vi "configureForVoltageOutput.vi"(2 "error in (no error)":errorcluster, 3 "Output Properties":T1, 4 "AnalogOutput in":refnum<class "AnalogOutput.lvclass">) -> (0 "error out":errorcluster, 1 "AnalogOutput out":refnum<class "AnalogOutput.lvclass">)   [LabVIEW 2011, in "Hardware.lvlib" / "Channels.lvlib" / "AnalogOutput.lvclass"]
doc: "Abstract Method.\n\nThis vi set the channel name, physical channel, and the output range of the DAC. It calls createChannel which is implemented by child classes (for example, niDAQmxAO).\n\nThe cluster passed to this vi includes:\n1) Name (string)\n2) Channels (String)\n3) Ranges (Double Array 1D)"
uses:
  AnalogOutput.lvclass
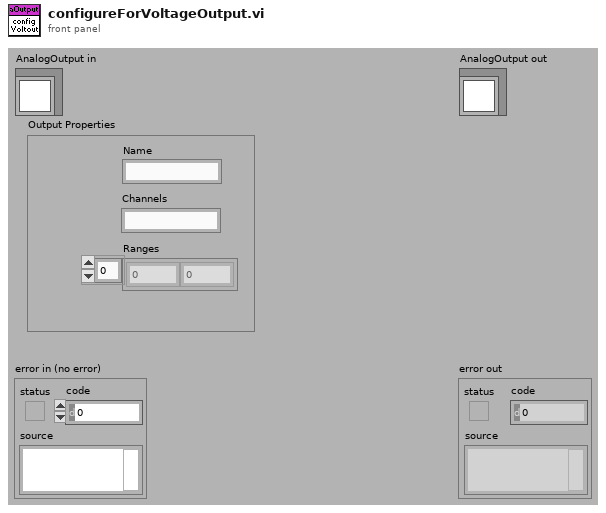
[diagram p1: front panel]
types:
  T1 = cluster{"Name":string, "Channels":string, "Ranges":dbl[]}
  T2 = cluster{"Configuration Type":cluster{"Differential":i16, "Pseudodifferential":i16, "RSE":dbl}, "Output Type":cluster{"Voltage":string, "Current":string, "Standard Function ":cluster{"Sine":string, "Square":string, "Triangle":string}}}
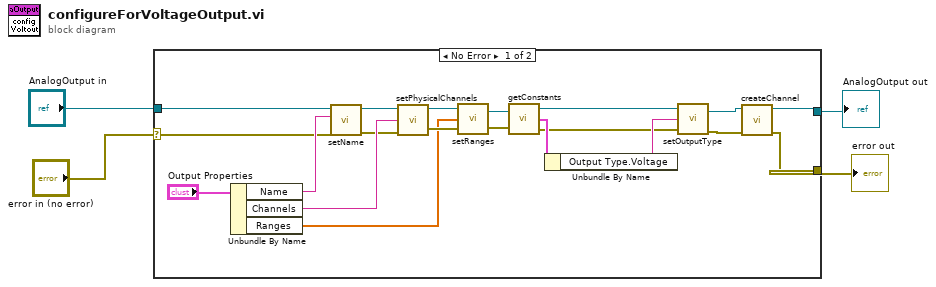
[diagram p0: block diagram]
diagram:
  n1 = case shown="No Error" "error in (no error)" {
    selector: "error in (no error)" -> [w21 w26]
    tunnel: [w8 w26] -> w3
    tunnel: [w7 w25] -> w1
    tunnel: "AnalogOutput in" -> [w23 w25]
    frame No Error {
      n2 = Unbundle By Name("Output Properties") -> ("Name"=w22:string, "Channels"=w19:string, "Ranges"=w5:dbl[])
      n3 = call "setName.vi"("error in (no error)"=w21, "name"=w22, "AnalogOutput.lvclass in"=w23) -> ("error out"=w18:errorcluster, "AnalogOutput.lvclass out"=w20:refnum<class "AnalogOutput.lvclass">)  [unwired: 7 in]
      n4 = call-dynamic "setPhysicalChannels.vi"("error in (no error)"=w18, "Physical Channels"=w19, "AnalogOutput.lvclass in"=w20) -> ("error out"=w16:errorcluster, "AnalogOutput.lvclass out"=w17:refnum<class "AnalogOutput.lvclass">)
      n5 = call "setRanges.vi"("error in (no error)"=w16, "Ranges"=w5, "AnalogOutput.lvclass in"=w17) -> ("error out"=w14:errorcluster, "AnalogOutput.lvclass out"=w15:refnum<class "AnalogOutput.lvclass">)
      n6 = call-dynamic "getConstants.vi"("AnalogOutput in"=w15, "error in (no error)"=w14) -> ("AnalogOutput out"=w11:refnum<class "AnalogOutput.lvclass">, "Constants"=w13:T2, "error out"=w10:errorcluster)
      n7 = Unbundle By Name(w13) -> ("Output Type.Voltage"=w12:string)
      n8 = call "setOutputType.vi"("error in (no error)"=w10, "Output Type"=w12, "AnalogOutput in"=w11) -> ("error out"=w6:errorcluster, "AnalogOutput out"=w9:refnum<class "AnalogOutput.lvclass">)
      n9 = call-dynamic "createChannel.vi"("error in (no error)"=w6, "AnalogOutput in"=w9) -> ("error out"=w8:errorcluster, "AnalogOutput out"=w7:refnum<class "AnalogOutput.lvclass">)  [unwired: 8 in]
    }
    frame Error {
    }
  }
  "error out" <- w3
  "AnalogOutput out" <- w1
